vi "Write Power.vi"(8 "error in (no error)":errorcluster, 10 "Power":bool, 11 "Control-Server in":refnum<class "Control-Server.lvclass">) -> (0 "error out":errorcluster, 3 "Control-Server out":refnum<class "Control-Server.lvclass">)   [LabVIEW 2015, in "Control-Server.lvclass"]
uses:
  Control-Server.lvclass
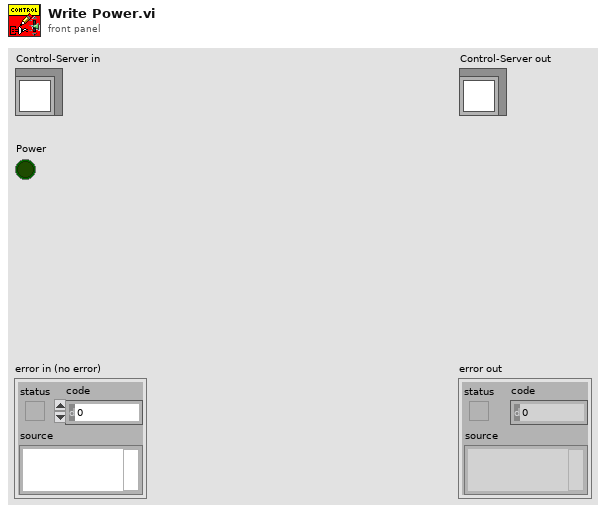
[diagram p1: front panel]
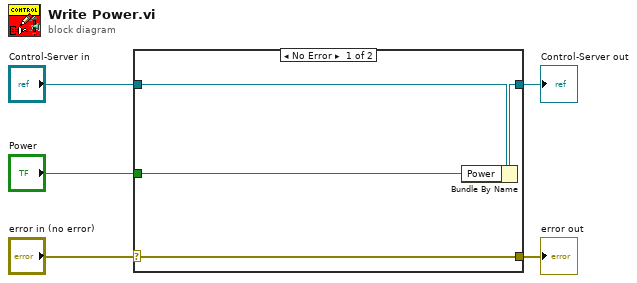
[diagram p0: block diagram]
diagram:
  n1 = case shown="No Error" "error in (no error)" {
    selector: "error in (no error)" -> [w9 w10]
    tunnel: [w9 w10] -> w4
    tunnel: [w7 w11] -> w2
    tunnel: "Control-Server in" -> [w8 w11]
    tunnel: "Power" -> [w6 _]
    frame No Error {
      n2 = Bundle By Name(cluster=w8, "Power"=w6) -> (w7:refnum<class "Control-Server.lvclass">)
    }
    frame Error {
    }
  }
  "error out" <- w4
  "Control-Server out" <- w2
